vi "DisplayDeviceInfo.vi"(3 "error in":errorcluster, 4 "DevInfoList In":refnum<k24>, 5 "Output Refnum In":refnum<vi>) -> (0 "error out":errorcluster, 1 "DevInfoList Out":refnum<k24>, 2 "Output Refnum Out":refnum<vi>)   [LabVIEW 2009]
uses:
  C:/Samples/LabVIEW/UseUSBAddress/LabVIEW 2009/UsbDllWrap.dll
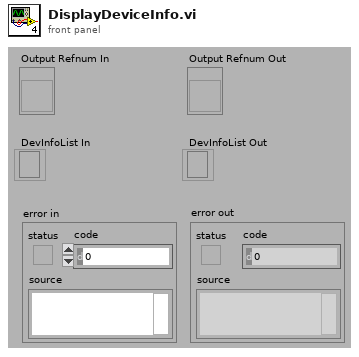
[diagram p1: front panel]
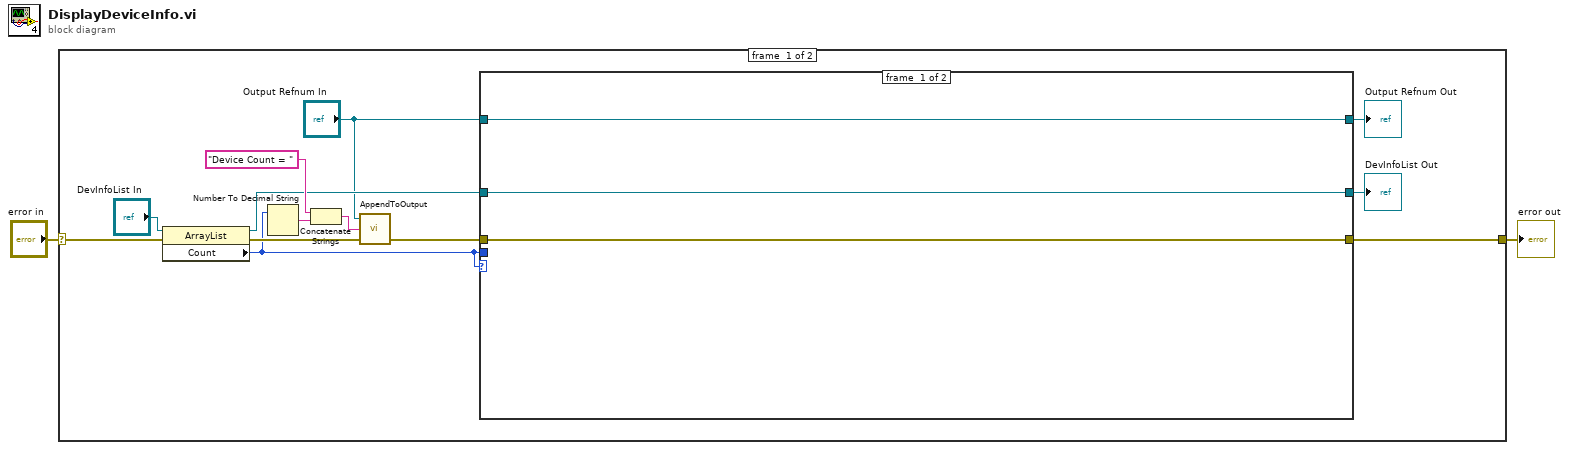
[diagram p0: block diagram]
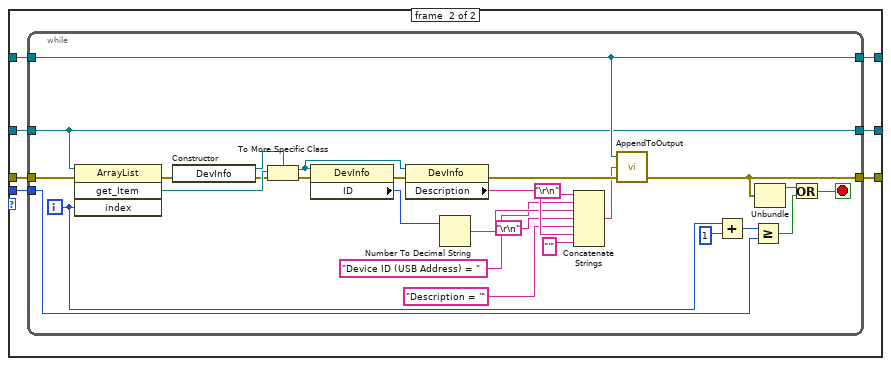
[diagram p2: hidden frame]
diagram:
  n1 = case shown="No Error" "error in" {
    selector: "error in" -> [w4 w54]
    tunnel: [w8 w54] -> w2
    frame #0 {
      n2 = property class="ArrayList"(reference="DevInfoList In", error in=w4) -> (reference out=w10:refnum<k24>, error out=w11:errorcluster, "Count"=w3:i32)
      n3 = Number To Decimal String(number=w3) -> (decimal integer string=w15:string)  [unwired: 1 in]
      n4 = Concatenate Strings("Device Count = ", w15) -> (w13:string)
      n5 = call "AppendToOutput.vi"("error in"=w11, "Input String"=w13, "Output Refnum In"="Output Refnum In") -> ("error out"=w9:errorcluster)  [unwired: 1 in, 1 out]
      n6 = case shown="1, Default" w3 {
        tunnel: w10 -> [w18 w25]
        tunnel: w9 -> [w17 w24]
        tunnel: w3 -> [_ w23]
        tunnel: [w17 w22] -> w8
        tunnel: [w16 w21] -> w7
        tunnel: [w18 w20] -> w6
        tunnel: "Output Refnum In" -> [w16 w19]
        frame #0 {
        }
        frame #1 {
          n7 = while {
            tunnel: w19 -> [w30]
            tunnel: w25 -> [w29]
            tunnel: w24 -> [w36]
            tunnel: w23 -> [w35]
            tunnel: [w31] -> w22
            tunnel: [w30] -> w21
            tunnel: [w29] -> w20
            i -> [w26]
            stop <- w34 stop-if-true
            n8 = invoke class="ArrayList" method="get_Item"(reference=w29, error in=w36, "index"=w26) -> (error out=w38:errorcluster, "get_Item"=w40:refnum<k24>)  [unwired: 1 in, 2 out]
            n9 = constructor class="DevInfo"(error in=w38) -> (reference out=w39:refnum<k24>, error out=w37:errorcluster)  [unwired: 2 in, 1 out]
            n10 = To More Specific Class(target class=w39, reference=w40, error in=w37) -> (specific class reference=w41:refnum<k24>, error out=w51:errorcluster)
            n11 = property class="DevInfo"(reference=w41, error in=w51) -> (error out=w52:errorcluster, "ID"=w42:i32)  [unwired: 1 out]
            n12 = property class="DevInfo"(reference=w41, error in=w52) -> (error out=w53:errorcluster, "Description"=w49:string)  [unwired: 1 out]
            n13 = Number To Decimal String(number=w42) -> (decimal integer string=w45:string)  [unwired: 1 in]
            n14 = Concatenate Strings("\r\n", "Device ID (USB Address) = ", w45, "\r\n", "Description = '", w49, "'") -> (w50:string)
            n15 = call "AppendToOutput.vi"("error in"=w53, "Input String"=w50, "Output Refnum In"=w30) -> ("error out"=w31:errorcluster)  [unwired: 1 in, 1 out]
            n16 = Add(x=w26, y=1) -> (x+y=w28:i32)
            n17 = Greater Or Equal?(x=w28, y=w35) -> (x >= y?=w32:bool)
            n18 = Unbundle(w31) -> ("status"=w33:bool)  [unwired: 2 out]
            n19 = Or(x=w33, y=w32) -> (x .or. y?=w34:bool)
          }
        }
      }
      "Output Refnum Out" <- w7
      "DevInfoList Out" <- w6
    }
    frame #1 {
    }
  }
  "error out" <- w2
